vi "Graphics-Create XY Cluster (1D).vi"(2 "Array":dbl[](array[numeric]), 3 "dx":dbl) -> (0 "XY cluster":cluster{"Array":dbl[], "Array":dbl[]})   [LabVIEW 2020]
uses:
  Math VIs/LinSpace (x0-dx-npts).vi
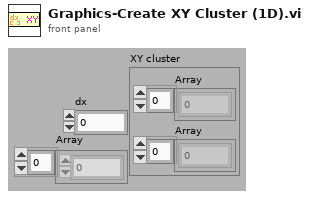
[diagram p1: front panel]
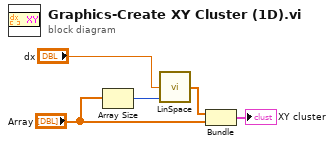
[diagram p0: block diagram]
diagram:
  n1 = Array Size(array="Array") -> (size(s)=w4:i32)
  n2 = call-poly "LinSpace.vi"("npts"=w4, "dx"="dx") -> ("Array"=w3:dbl[])  [unwired: 2 in, 1 out]
  n3 = Bundle("Array"=w3, "Array"="Array") -> (→"XY cluster":cluster{"Array":dbl[], "Array":dbl[]})  [unwired: 1 in]
